vi "IMIC_SetFilterChangerPosAbs.vi"(2 "Filter":i32, 3 "index":i32, 4 "handle":u64) -> (0 "handle out":u64, 1 "output param":T1(ring))   [LabVIEW 2011]
uses:
  tillimic32.dll
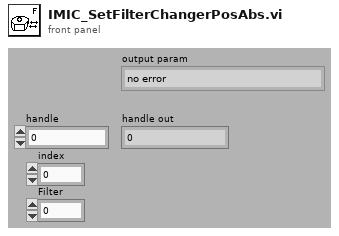
[diagram p1: front panel]
types:
  T1 = enum16{"no error", "missing axis", "missing Z axis", "missing Filter", "iMic not initialized", "no property", "wrong handle", "protocol not finished", "user parameter to long (>32 bits)", "no user parameter handle", "failed to open comport", "failed to initialize"}
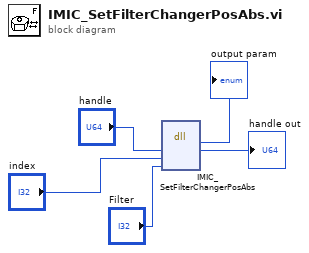
[diagram p0: block diagram]
diagram:
  n1 = dll-call lib="D:/Colibri/Drivers/TILLPhotonics/tillimic*.*" fn="IMIC_SetFilterChangerPosAbs"("handle"="handle", "index"="index", "Filterpos"="Filter") -> ("return type"=→"output param":i32, "handle"=→"handle out":u64)  [unwired: 5 in, 2 out]
